vi "Dual_Joy_Ctrl.vi"(8 "Joy1_1(Y)":dbl, 9 "Joy1_0(X)":dbl, 10 "Joy0_1(Y)":dbl, 11 "Joy0_0(X)":dbl) -> (1 "Z":dbl, 2 "Y":dbl, 3 "X":dbl)   [LabVIEW 2017]
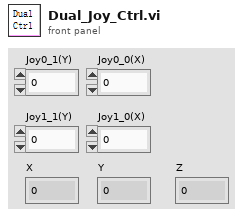
[diagram p1: front panel]
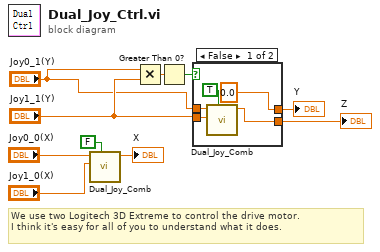
[diagram p0: block diagram]
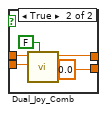
[diagram p2: hidden frame]
diagram:
  # "We use two Logitech 3D Extreme to control the drive motor.\nI think it's easy for all of you to understand what it does."
  n1 = call "Dual_Joy_Comb.vi"("Rotation"=FALSE, "Joy2"="Joy1_0(X)", "Joy1"="Joy0_0(X)") -> ("Output"=→"X":dbl)  [unwired: 8 in]
  n2 = Multiply(x="Joy0_1(Y)", y="Joy1_1(Y)") -> (x*y=w7:dbl)
  n3 = Greater Than 0?(x=w7) -> (x > 0?=w8:bool)
  n4 = case shown="False" w8 {
    tunnel: "Joy1_1(Y)" -> [w12 w18]
    tunnel: "Joy0_1(Y)" -> [w13 w19]
    tunnel: [0.0 w17] -> w6
    tunnel: [w11 0.0] -> w5
    frame False {
      n5 = call "Dual_Joy_Comb.vi"("Rotation"=TRUE, "Joy2"=w12, "Joy1"=w13) -> ("Output"=w11:dbl)  [unwired: 8 in]
    }
    frame True {
      n6 = call "Dual_Joy_Comb.vi"("Rotation"=FALSE, "Joy2"=w18, "Joy1"=w19) -> ("Output"=w17:dbl)  [unwired: 8 in]
    }
  }
  "Y" <- w6
  "Z" <- w5
